vi "Try Reconnect.vi"(8 "error in (no error)":errorcluster, 11 "IP Connection in":refnum<class "IP Connection.lvclass">) -> (0 "error out":errorcluster, 3 "IP Connection out":refnum<class "IP Connection.lvclass">)   [LabVIEW 2011, in "Tinkerforge.lvlib" / "IP Connection.lvclass"]
doc: "This VI tries to reconnect to the target address and port if necessary."
uses:
  IP Connection.lvclass
  Type Definitions/Connection Status.ctl
  IP Connection.lvclass/IP Connection.ctl
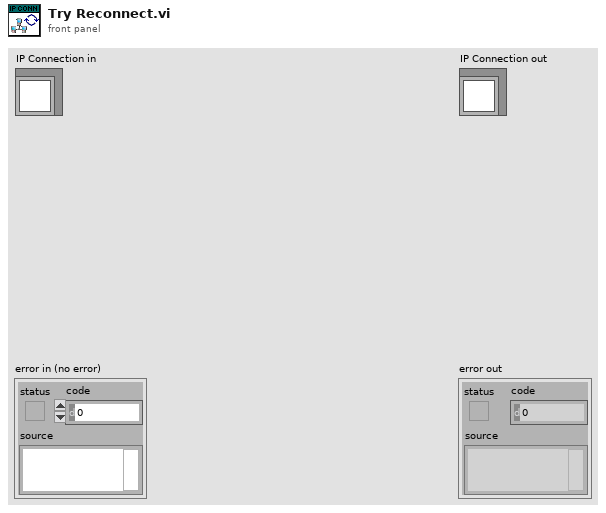
[diagram p1: front panel]
types:
  T1 = typedef "Tinkerforge.lvlib/IP Connection.lvclass/Connection Status.ctl" = enum16{"Uninitialized", "Connected", "Reconnecting", "Disconnected"}
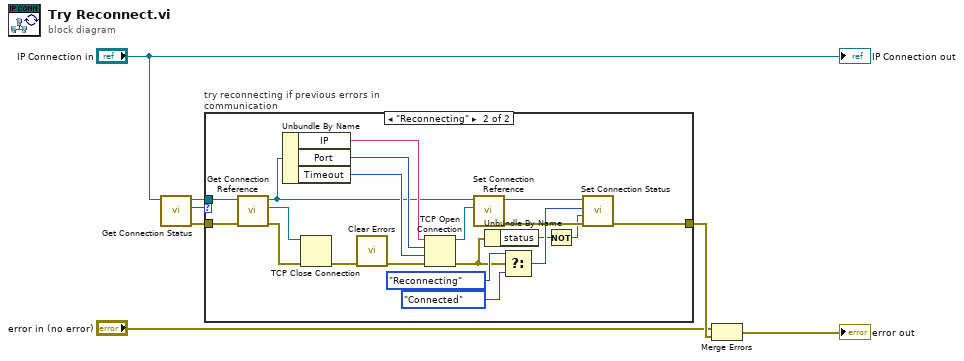
[diagram p0: block diagram]
diagram:
  n1 = call "Get Connection Status.vi"("IP Connection in"="IP Connection in") -> ("error out"=w4:errorcluster, "Connection Status"=w6:T1, "IP Connection out"=w5:refnum<class "IP Connection.lvclass">)  [unwired: 7 in, 1 out]
  n2 = case "try reconnecting if previous errors in communication" shown="\"Reconnecting\"" w6 {
    tunnel: w5 -> [_ w27]
    tunnel: w4 -> [w8 w28]
    tunnel: [w8 w9] -> w3
    frame Default {
    }
    frame "Reconnecting" {
      n3 = call "Get Connection Reference.vi"("error in (no error)"=w28, "IP Connection in"=w27) -> ("error out"=w25:errorcluster, "TCP Network Connection"=w26:refnum<k5>, "IP Connection out"=w19:refnum<class "IP Connection.lvclass">)  [unwired: 7 in]
      n4 = Unbundle By Name(w19) -> ("IP"=w22:string, "Port"=w21:u16, "Timeout"=w20:i32)
      n5 = TCP Close Connection(connection ID=w26, error in (no error)=w25) -> (error out=w24:errorcluster)  [unwired: 1 in, 1 out]
      n6 = call <vilib>:"Clear Errors.vi"("error in (no error)"=w24) -> ("error out"=w23:errorcluster)  [unwired: 6 in]
      n7 = TCP Open Connection(address=w22, remote port or service name=w21, timeout ms (60000)=w20, error in (no error)=w23) -> (connection ID=w17:refnum<k5>, error out=w12:errorcluster)  [unwired: 1 in]
      n8 = call "Set Connection Reference.vi"("TCP Network Connection"=w17, "IP Connection in"=w19) -> ("error out"=w16:errorcluster, "IP Connection out"=w18:refnum<class "IP Connection.lvclass">)  [unwired: 8 in]
      n9 = Unbundle By Name(w12) -> ("status"=w11:bool)
      n10 = Select(t=Connection_Status."Reconnecting" ("Connection Status"), s=w12, f=Connection_Status."Connected" ("Connection Status")) -> (s? t:f=w13:T1)
      n11 = Not(x=w11) -> (.not. x?=w10:bool)
      n12 = call "Set Connection Status.vi"("error in (no error)"=w16, "connected?"=w10, "Connection Status"=w13, "IP Connection in"=w18) -> ("error out"=w9:errorcluster)  [unwired: 6 in, 1 out]
    }
  }
  n13 = Merge Errors("error in (no error)", w3) -> (→"error out":errorcluster)
  "IP Connection out" <- "IP Connection in"
